vi "Termo_1.5__.vi"() -> ()   [LabVIEW 2015]
doc: "Программа мониторинга температуры"
uses:
  <vilib>/Utility/error.llb/DialogType.ctl
  Load and Save Controls_LV2009.llb/RWC_Actions.ctl
panel:
  out "?":bool
  out "graph_update":bool
  out "Конфиг. АЦП?":bool
  in  "Tab Control":enum32{"ИЗМЕРЕНИЯ [К]", " АЦП", "ГРАФИК"}(tab)
  in  "T2_visible":bool=TRUE
  out "T6":dbl format="%.2f"
  in  "T5_visible":bool=TRUE
  out "R5":dbl format="%.2f"
  out "T5":dbl format="%.2f"
  out "R1":dbl format="%.2f"
  out "T1":dbl format="%.2f"
  out "T3":dbl format="%.2f"
  out "R3":dbl format="%.2f"
  out "Alarm":bool
  out "разница Т":dbl format="%.2f"
  out "T2":dbl format="%.2f"
  out "T4":dbl format="%.2f"
  out "R2":dbl format="%.2f"
  out "R4":dbl format="%.2f"
  out "R6":dbl format="%.2f"
  in  "T1_visible":bool=TRUE
  in  "T3_visible":bool=TRUE
  in  "T4_visible":bool=TRUE
  in  "T6_visible":bool=TRUE
  in  "stop":bool
  in  "ADC_dyn_range":T1(ring)=enum."± 0.625 В"
  in  "Buf_size":u8=1 min=1 max=128
  in  "SPS":T2(ring)
  in  "IP-адрес":string="192.168.127.252"
  in  "порт":u16=4001
  in  "Очистить график":bool
  in  "load_coeff.":bool caption="Disconn"
  in  "save_coeff.":bool caption="Disconn"
  in  "Coeff_cl_ch5":T3={"k1"=19.4736079181311652, "k2"=-232.79779903171584, "k3"=1229.13228608109057005, "k4"=-3103.0388431325554801, "k5"=4219.3520172238349901, "k6"=-2697.7160155214369299, "k7"=779.55193291697651198} caption="Канал 5" {"k7" format="%#_16g"; "k6" format="%#_16g"; "k5" format="%#_16g"; "k4" format="%#_16g"; "k3" format="%#_16g"; "k2" format="%#_16g"; "k1" format="%#_16g"}
  in  "Coeff_cl_ch4":T3={"k1"=24.218377729237545301, "k2"=-311.679773783311248, "k3"=1734.44359050504863, "k4"=-4665.87189712375402, "k5"=6719.3289510309696202, "k6"=-4578.02570509165525, "k7"=1400.00134176202118} caption="Канал 4" {"k7" format="%#_16g"; "k6" format="%#_16g"; "k5" format="%#_16g"; "k4" format="%#_16g"; "k3" format="%#_16g"; "k2" format="%#_16g"; "k1" format="%#_16g"}
  in  "Coeff_cl_ch3":T3={"k1"=8.756, "k2"=-142.210000000000000006, "k3"=1253.0, "k4"=-4877.1, "k5"=10581.0, "k6"=-10354.0, "k7"=3998.5} caption="Канал 3" {"k7" format="%#_16g"; "k6" format="%#_16g"; "k5" format="%#_16g"; "k4" format="%#_16g"; "k3" format="%#_16g"; "k2" format="%#_16g"; "k1" format="%#_16g"}
  in  "Coeff_cl_ch2":T3={"k1"=31.9101907935109921, "k2"=-399.867376562207937, "k3"=2119.32627579197288, "k4"=-5531.15447566658258, "k5"=7772.21873644739389, "k6"=-5292.23886113613844, "k7"=1613.2211984321475} caption="Канал 2" {"k7" format="%#_16g"; "k6" format="%#_16g"; "k5" format="%#_16g"; "k4" format="%#_16g"; "k3" format="%#_16g"; "k2" format="%#_16g"; "k1" format="%#_16g"}
  in  "Coeff_cl_ch6":T3={"k1"=11.9061392787261866, "k2"=-139.902402561856434, "k3"=774.882810204289854, "k4"=-1837.4832512177527, "k5"=2139.5822282396256899, "k6"=-730.555961686186492, "k7"=169.810834781266749} caption="Канал 6" {"k7" format="%#_16g"; "k6" format="%#_16g"; "k5" format="%#_16g"; "k4" format="%#_16g"; "k3" format="%#_16g"; "k2" format="%#_16g"; "k1" format="%#_16g"}
  in  "GraphLookB":bool
  in  "xScale -":bool
  in  "xScale +":bool
  out "мин.":string="1"
  in  "Старт измер.":bool
  in  "Стоп измер.":bool
  in  "Добавить время":dbl(ring)=300.0 items=["10 сек."=10.0, "1 мин."=60.0, "5 мин."=300.0, "20 мин."=1200.0]
  in  "Т min":dbl=4.0 min=-10.0 max=350.0 step=0.1
  in  "Т max":dbl=300.0 min=2.0 max=500.0 step=0.1
  out "часы":string="0"
  in  "Autoscale":bool=TRUE
  out "сек.":string="0"
  out "Сутки":string
  out "счетчик":u32=4001
  in  "Запись в файл":bool
  out "Path":string
  out "refnum out":refnum<file>
  in  "header?":bool caption="Disconn"
  out "con ID":refnum<k5>
  out "Graphs T":dynamicdata(graph) caption="ТЕМПЕРАТУРА, К"
  out "Расположение файла":path
  # "Конец  соленоида"
  # "Середина\n соленоида"
  # "Перемычка"
  # "Кольцо\n спаев 1"
  # "Кольцо\n спаев 2"
  # "Шина"
  # "Конец сол/спаи dT:"
  # "Больше 40 К ?"
  # "Сопротивление, Ом"
  # "Конец соленоида"
  # "Сер. соленоида"
  # "Перемычка"
  # "1"
  # "Кольцо спаев"
  # "2"
  # "Шина"
  # "Скорость измерений"
  # "SPS = Samples Per Second"
  # "Размер буфера усреднения"
  # "Подключение"
  # "Шкала Т"
  # "Время графика"
  # ":"
  # ":"
  # "Измерения"
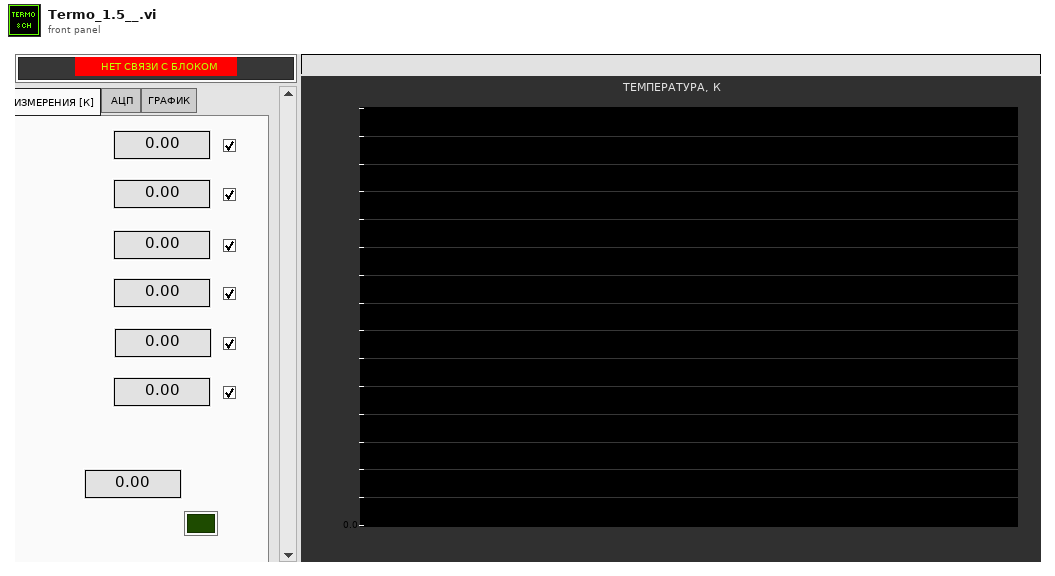
[diagram p1: front panel]
types:
  T1 = enum16{"± 5 В", "± 2.5 В", "± 1.25 В", "± 0.625 В", "± 312.5 мВ", "± 156.25 мВ", "± 78.125 мВ"}
  T2 = enum16{"2,5 SPS", "5 SPS", "10 SPS", "25 SPS", "50 SPS", "100 SPS", "500 SPS"}
  T3 = cluster{"k1":ext, "k2":ext, "k3":ext, "k4":ext, "k5":ext, "k6":ext, "k7":ext}
  T4 = typedef "RWC_Actions.ctl" = enum16{"Read", "Write", "Read and Create"}
  T5 = typedef "DialogType.ctl" = u16
  T6 = enum32{"Page Enabled", "Page Disabled", "Page Disabled & Grayed"}
  T7 = enum16{"Standard", "Buffered", "CRLF", "Immediate"}
  T8 = cluster{" T1":dbl, "T2":dbl, "T3":dbl, "T4":dbl, " T5":dbl, "T6":dbl}
  T9 = typedef "LVDateTimeRec.ctl" = cluster{"fractional second":dbl, "second":i32, "minute":i32, "hour":i32, "day of month":i32, "month":i32, "year":i32, "day of week":i32, "day of year":i32, "DST":i32}
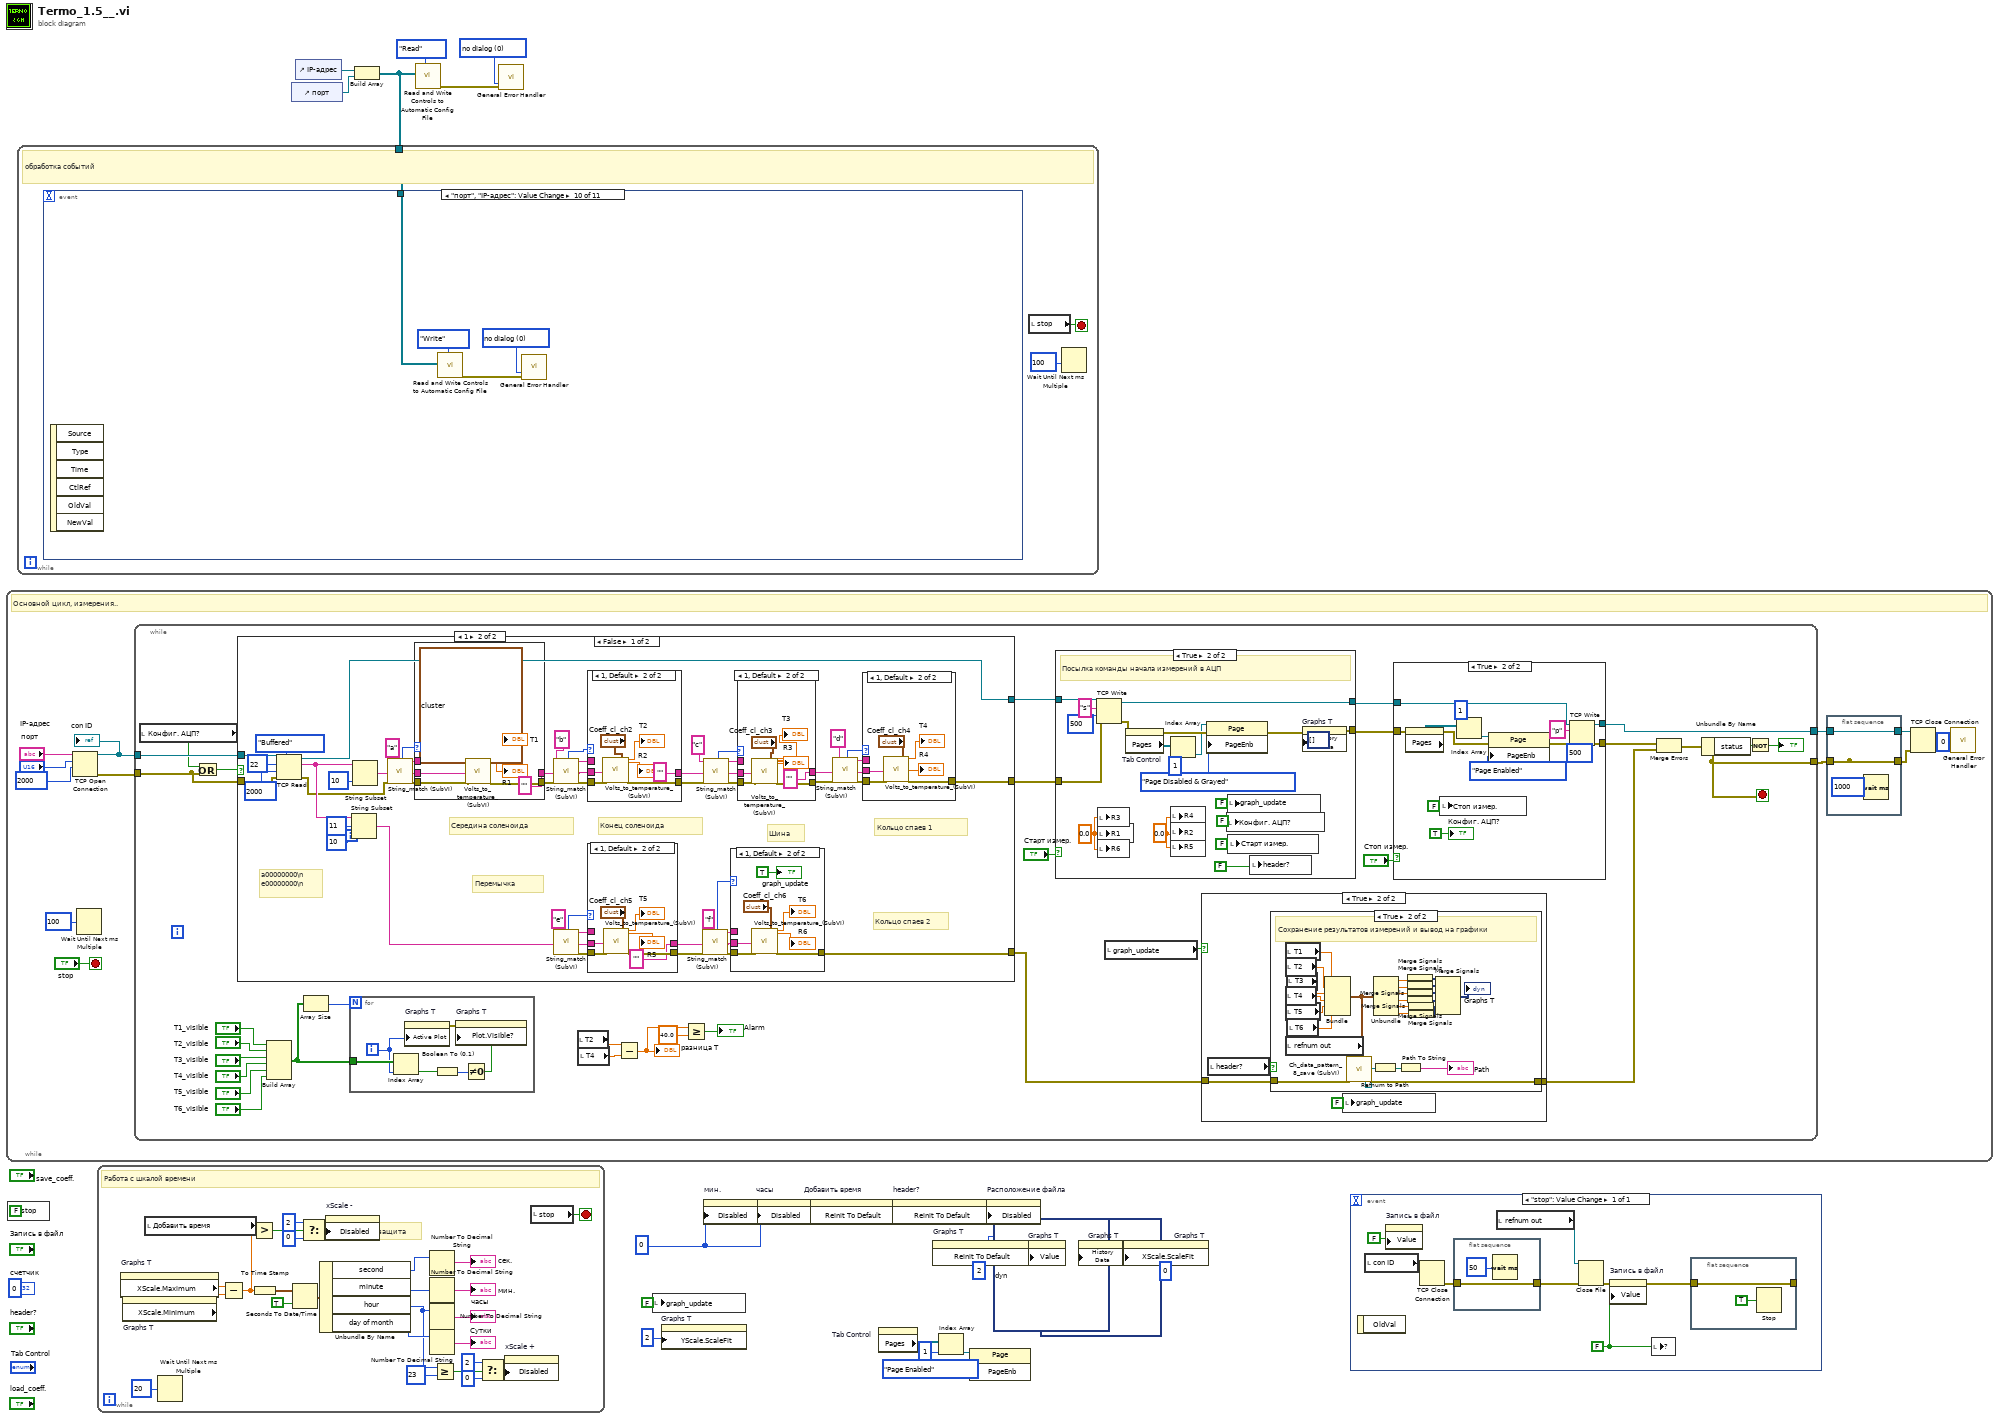
[diagram p0: block diagram]
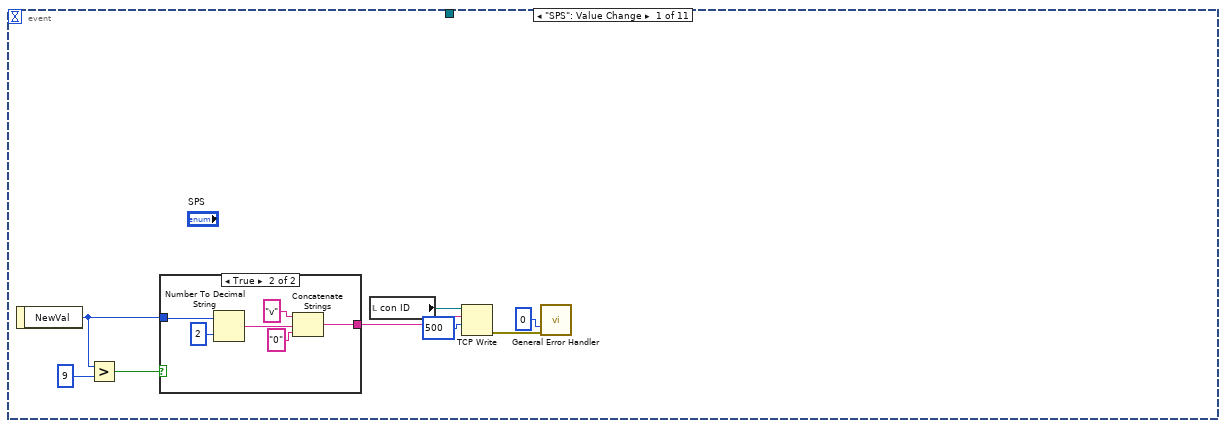
[diagram p2: hidden frame]
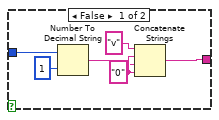
[diagram p3: hidden frame]
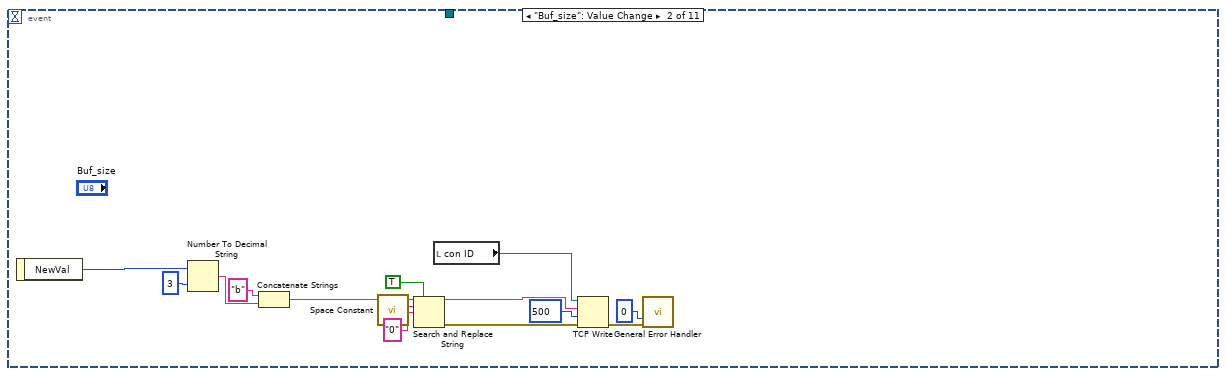
[diagram p4: hidden frame]
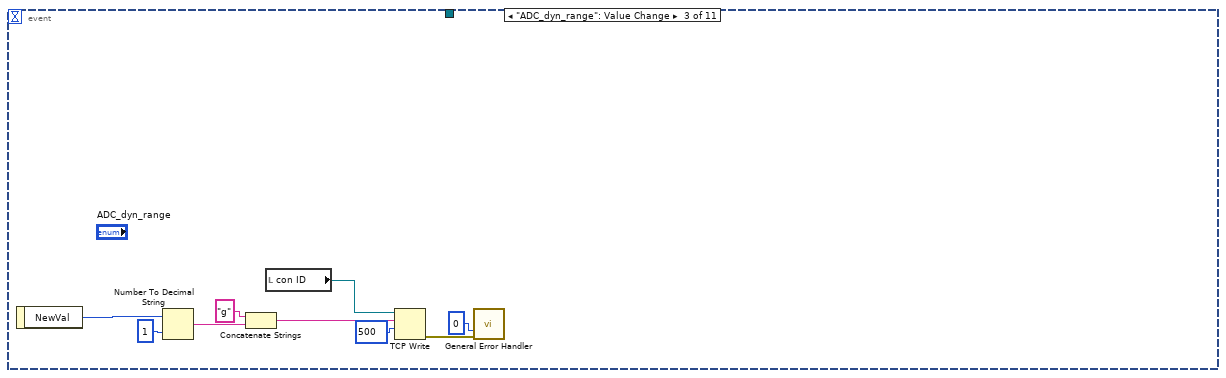
[diagram p5: hidden frame]
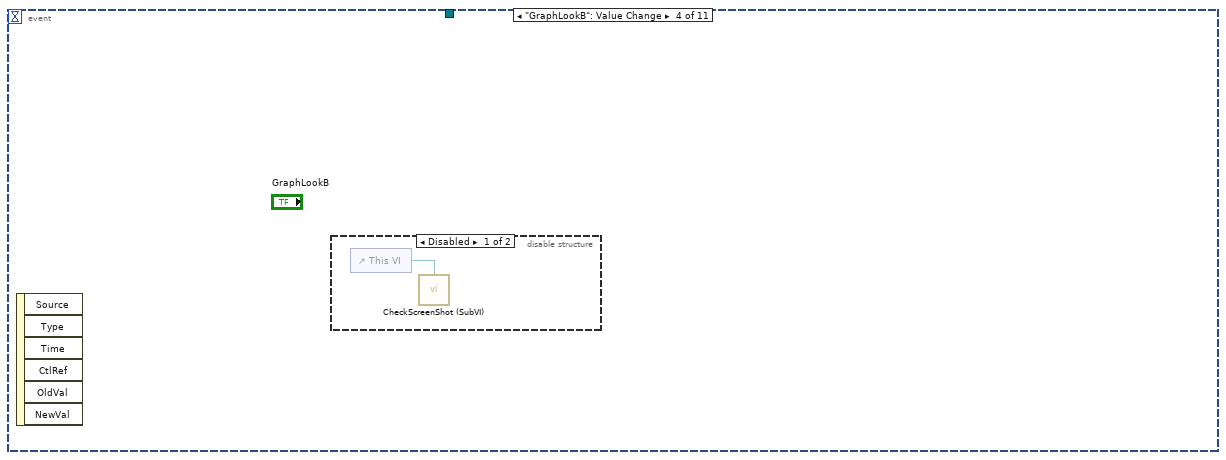
[diagram p6: hidden frame]
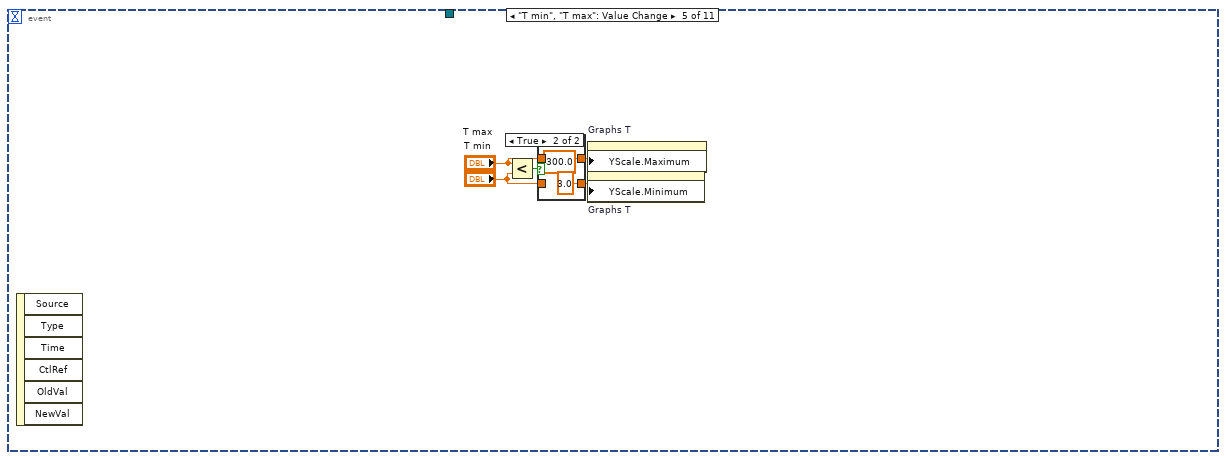
[diagram p8: hidden frame]
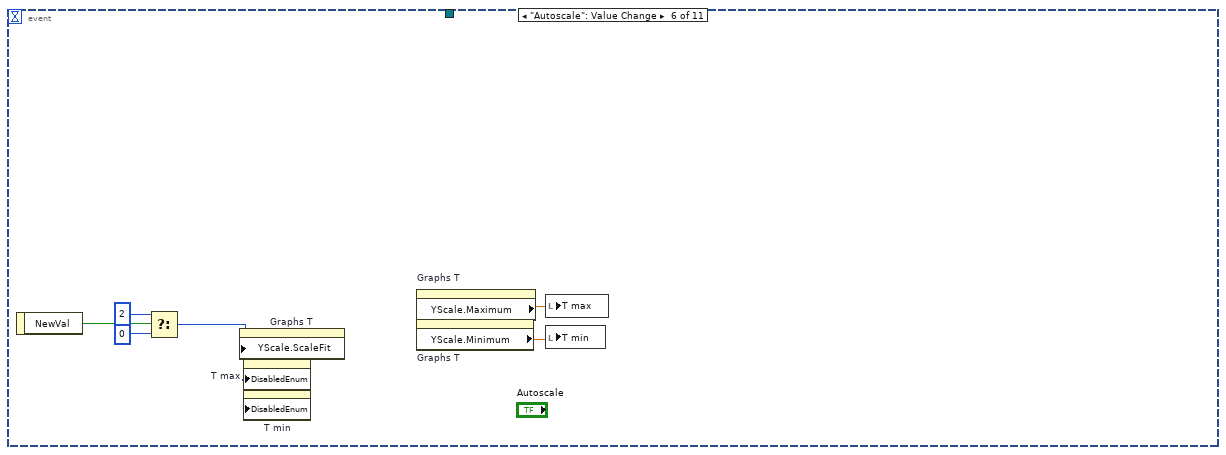
[diagram p10: hidden frame]
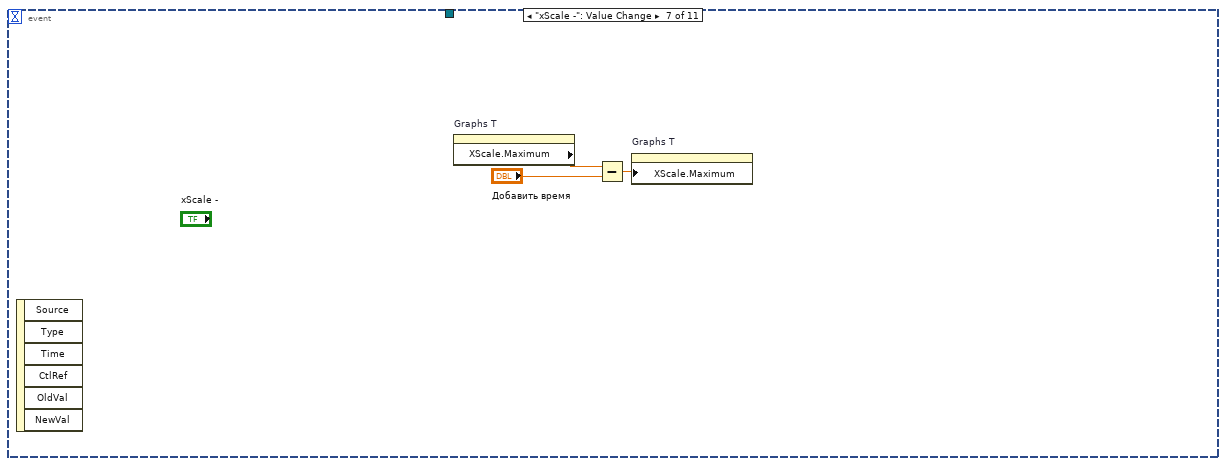
[diagram p11: hidden frame]
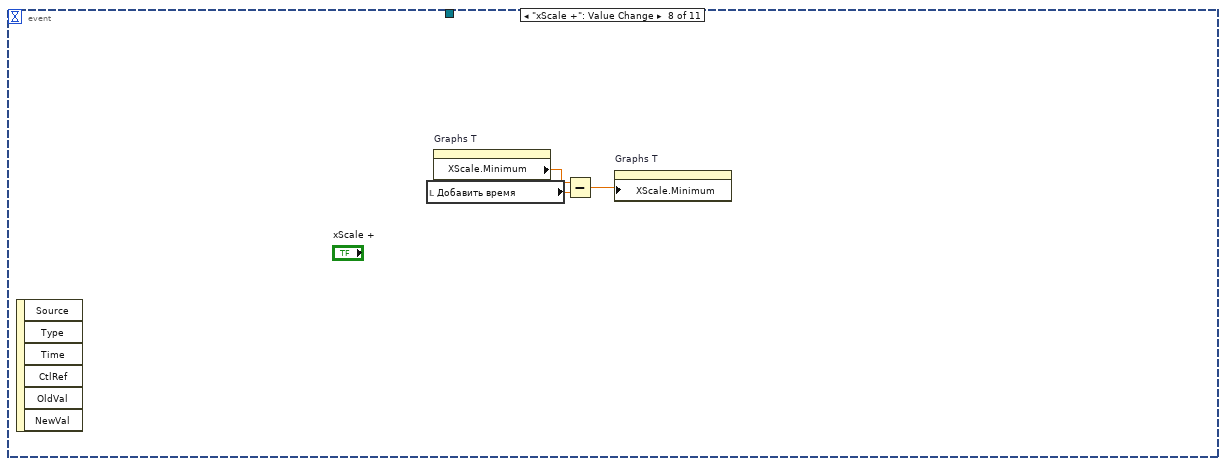
[diagram p12: hidden frame]
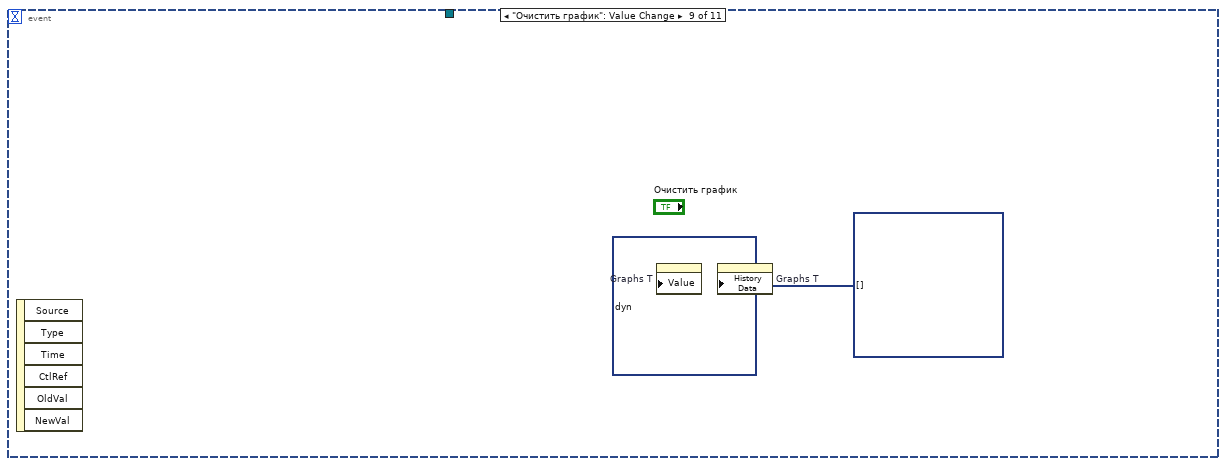
[diagram p13: hidden frame]
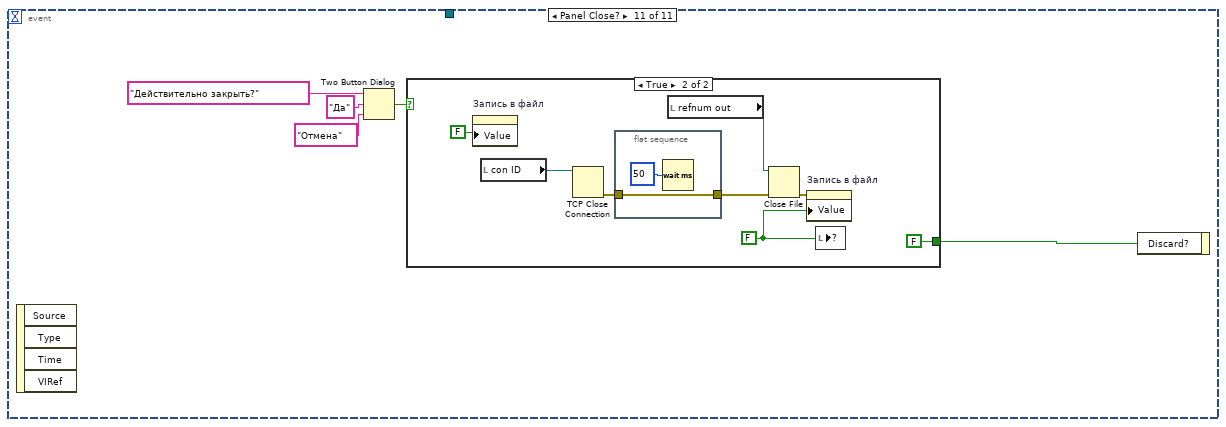
[diagram p14: hidden frame]
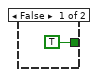
[diagram p15: hidden frame]
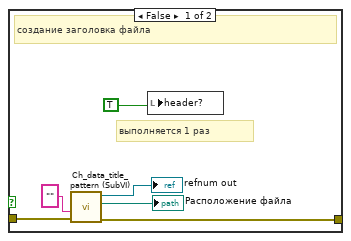
[diagram p17: hidden frame]
diagram:
  w6 = T5 0 items=["no dialog", "OK message", "continue or stop message", "OK message + warnings", "continue/stop + warnings"] ("type of dialog (OK msg:1)")
  w25 = u8 0 ("Disabled")
  n1 = while {
    stop <- "stop" stop-if-true
    # "Основной цикл, измерения.."
    n2 = TCP Open Connection(address="IP-адрес", remote port or service name="порт", timeout ms (60000)=2000) -> (connection ID=w38:refnum<k5>, error out=w32:errorcluster)  [unwired: 1 in, 1 out]
    "con ID" <- w38
    n3 = Wait Until Next ms Multiple(millisecond multiple=u32 100) -> ()  [unwired: 1 out]
    n4 = while {
      tunnel: w38 -> [w73]
      tunnel: w32 -> [w51]
      tunnel: [w44] -> w30
      tunnel: [w43] -> w28
      stop <- w43 stop-if-true
      n5 = local read "Конфиг. АЦП?"() -> (w52:bool)
      n6 = Or(x=w52, y=w51) -> (x .or. y?=w66:bool)
      n7 = case shown="False" w66 {
        tunnel: [w156 w259] -> w53
        tunnel: w73 -> [w159 w259]
        tunnel: [w155 w258] -> w49
        tunnel: w51 -> [w157 w258]
        tunnel: [w154 _] -> w47
        frame False {
          # "a00000000\\n\ne00000000\\n"
          # "Кольцо спаев 2"
          # "Шина"
          # "Перемычка"
          # "Кольцо спаев 1"
          # "Конец соленоида"
          # "Середина соленоида"
          n8 = TCP Read(connection ID=w159, bytes to read=22, error in (no error)=w157, 7:T7."Buffered" ("mode (standard)"), 9:2000 ("timeout ms (25000)")) -> (connection ID out=w156:refnum<k5>, data out=w163:string, error out=w158:errorcluster)
          n9 = String Subset(string=w163, offset (0)=11, length (rest)=10 ("length (rest)")) -> (substring=w160:string)
          n10 = String Subset(string=w163, length (rest)=10 ("length (rest)")) -> (substring=w165:string)  [unwired: 1 in]
          n11 = call "String_match (SubVI).vi"("channel id"="a" ("regular expression"), "input string"=w165, "error in"=w158) -> ("match ?"=w171:i32, "output string"=w199:string, "match substring"=w200:string, "error out"=w201:errorcluster)  [unwired: 13 in]
          n12 = case shown="1" w171 {
            tunnel: [w250 w256] -> w190
            tunnel: w201 -> [w250 w257]
            tunnel: w200 -> [_ w252]
            tunnel: [w249 "" ("output string")] -> w203
            tunnel: w199 -> [w249 _]
            frame -1, Default {
            }
            frame 1 {
              n13 = call "Volts_to_temperature_(SubVI).vi"("ch_data_string"=w252, "error in"=w257, "koeff. cluster"=T3 {"k1"=20.678416953771299999, "k2"=-270.806564304511, "k3"=1559.71508308313, "k4"=-4317.07993103563, "k5"=6444.9990497231400002, "k6"=-4562.30018320679, "k7"=1455.99202726967}) -> ("T solvation"=→"T1":dbl, "meas_voltage"=→"R1":dbl, "error out"=w256:errorcluster)  [unwired: 20 in, 2 out]
            }
          }
          n14 = call "String_match (SubVI).vi"("channel id"="b" ("regular expression"), "input string"=w203, "error in"=w190) -> ("match ?"=w170:i32, "output string"=w195:string, "match substring"=w196:string, "error out"=w197:errorcluster)  [unwired: 13 in]
          n15 = call "String_match (SubVI).vi"("channel id"="e" ("regular expression"), "input string"=w160) -> ("match ?"=w167:i32, "output string"=w188:string, "match substring"=w187:string, "error out"=w186:errorcluster)  [unwired: 14 in]
          n16 = case shown="1, Default" w170 {
            tunnel: [w241 w248] -> w179
            tunnel: w197 -> [w241 w247]
            tunnel: w196 -> [_ w246]
            tunnel: w195 -> [w240 _]
            tunnel: [w240 "" ("output string")] -> w178
            frame -1 {
            }
            frame 1, Default {
              n17 = call "Volts_to_temperature_(SubVI).vi"("ch_data_string"=w246, "error in"=w247, "koeff. cluster"="Coeff_cl_ch2") -> ("T solvation"=→"T2":dbl, "meas_voltage"=→"R2":dbl, "error out"=w248:errorcluster)  [unwired: 20 in, 2 out]
            }
          }
          n18 = case shown="1, Default" w167 {
            tunnel: [w225 w232] -> w189
            tunnel: w186 -> [w225 w231]
            tunnel: w187 -> [_ w230]
            tunnel: [w224 "" ("output string")] -> w184
            tunnel: w188 -> [w224 _]
            frame -1 {
            }
            frame 1, Default {
              n19 = call "Volts_to_temperature_(SubVI).vi"("ch_data_string"=w230, "error in"=w231, "koeff. cluster"="Coeff_cl_ch5") -> ("T solvation"=→"T5":dbl, "meas_voltage"=→"R5":dbl, "error out"=w232:errorcluster)  [unwired: 20 in, 2 out]
            }
          }
          n20 = call "String_match (SubVI).vi"("channel id"="f" ("regular expression"), "input string"=w184, "error in"=w189) -> ("match ?"=w166:i32, "output string"=w183:string, "match substring"=w182:string, "error out"=w181:errorcluster)  [unwired: 13 in]
          n21 = call "String_match (SubVI).vi"("channel id"="c" ("regular expression"), "input string"=w178, "error in"=w179) -> ("match ?"=w169:i32, "output string"=w174:string, "match substring"=w175:string, "error out"=w176:errorcluster)  [unwired: 13 in]
          n22 = case shown="1, Default" w166 {
            tunnel: [w216 w223] -> w154
            tunnel: w181 -> [w216 w222]
            tunnel: w182 -> [_ w221]
            tunnel: w183 -> [_ _]
            frame -1 {
            }
            frame 1, Default {
              n23 = call "Volts_to_temperature_(SubVI).vi"("ch_data_string"=w221, "error in"=w222, "koeff. cluster"="Coeff_cl_ch6") -> ("T solvation"=→"T6":dbl, "meas_voltage"=→"R6":dbl, "error out"=w223:errorcluster)  [unwired: 20 in, 2 out]
              "graph_update" <- TRUE ("graph_update")
            }
          }
          n24 = case shown="1, Default" w169 {
            tunnel: w176 -> [w208 w214]
            tunnel: [w208 w213] -> w173
            tunnel: w175 -> [_ w210]
            tunnel: w174 -> [w207 _]
            tunnel: [w207 "" ("output string")] -> w172
            frame -1 {
            }
            frame 1, Default {
              n25 = call "Volts_to_temperature_(SubVI).vi"("ch_data_string"=w210, "error in"=w214, "koeff. cluster"="Coeff_cl_ch3") -> ("T solvation"=→"T3":dbl, "meas_voltage"=→"R3":dbl, "error out"=w213:errorcluster)  [unwired: 20 in, 2 out]
            }
          }
          n26 = call "String_match (SubVI).vi"("channel id"="d" ("regular expression"), "input string"=w172, "error in"=w173) -> ("match ?"=w168:i32, "output string"=w191:string, "match substring"=w192:string, "error out"=w193:errorcluster)  [unwired: 13 in]
          n27 = case shown="1, Default" w168 {
            tunnel: w193 -> [w233 w239]
            tunnel: [w233 w238] -> w155
            tunnel: w192 -> [_ w236]
            tunnel: w191 -> [_ _]
            frame -1 {
            }
            frame 1, Default {
              n28 = call "Volts_to_temperature_(SubVI).vi"("ch_data_string"=w236, "error in"=w239, "koeff. cluster"="Coeff_cl_ch4") -> ("T solvation"=→"T4":dbl, "meas_voltage"=→"R4":dbl, "error out"=w238:errorcluster)  [unwired: 20 in, 2 out]
            }
          }
        }
        frame True {
        }
      }
      n29 = Build Array("T1_visible", "T2_visible", "T3_visible", "T4_visible", "T5_visible", "T6_visible") -> (w58:bool[])
      n30 = Array Size(array=w58) -> (size(s)=w59:i32)
      n31 = for {
        N: w59 -> [_]
        tunnel: w58 -> [w152]
        i -> [w150]
        n32 = Index Array(array=w152, index=w150) -> (element=w149:bool)
        n33 = property on="Graphs T" class="WFChart (strict)"("Active Plot"=w150) -> (error out=w151:errorcluster)  [unwired: 2 in, 1 out]
        n34 = Boolean To (0,1)(Boolean=w149) -> (0, 1=w153:i16)
        n35 = Not Equal To 0?(x=w153) -> (x != 0?=w148:bool)
        n36 = property on="Graphs T" class="WFChart (strict)"(error in=w151, "Plot.Visible?"=w148) -> ()  [unwired: 1 in, 2 out]
      }
      n37 = local read "T2"() -> (w68:dbl)
      n38 = local read "T4"() -> (w67:dbl)
      n39 = Subtract(x=w68, y=w67) -> (x-y=w69:dbl)
      "разница Т" <- w69
      n40 = Greater Or Equal?(x=w69, y=40.0) -> (x >= y?=→"Alarm":bool)
      n41 = case shown="True" "Старт измер." {
        tunnel: [w126 w137] -> w55
        tunnel: [w127 w136] -> w57
        tunnel: w53 -> [w127 w131]
        tunnel: w49 -> [w126 w130]
        frame False {
        }
        frame True {
          w133 = 0.0 ("3")
          w128 = 0.0 ("3")
          # "Посылка команды начала измерений в АЦП"
          n42 = TCP Write(connection ID=w131, data in="s", error in (no error)=w130, 9:500 ("timeout ms (25000)")) -> (connection ID out=w136:refnum<k5>, error out=w145:errorcluster)  [unwired: 1 out]
          n43 = local write "R3"(w128) -> ()
          n44 = local write "R1"(w128) -> ()
          n45 = local write "R6"(w128) -> ()
          n46 = property on="Tab Control" class="TabCtl (strict)"(error in=w145) -> (error out=w146:errorcluster, "Pages"=w141:refnum<vi>[])  [unwired: 1 in, 1 out]
          n47 = Index Array(array=w141, index=1) -> (element=w142:refnum<vi>)
          n48 = local write "R4"(w133) -> ()
          n49 = local write "R2"(w133) -> ()
          n50 = local write "R5"(w133) -> ()
          n51 = property class="Page"(reference=w142, error in=w146, "PageEnb"=T6."Page Disabled & Grayed" ("Page Enabled State")) -> (error out=w132:errorcluster)  [unwired: 1 out]
          n52 = local write "Конфиг. АЦП?"(FALSE ("Старт измер.")) -> ()
          n53 = local write "graph_update"(FALSE ("graph_update")) -> ()
          n54 = local write "Старт измер."(FALSE ("Старт измер.")) -> ()
          n55 = local write "header?"(FALSE ("flag1")) -> ()
          n56 = property on="Graphs T" class="WFChart (strict)"(error in=w132, "History Data"=dynamicdata[] []) -> (error out=w137:errorcluster)  [unwired: 1 in, 1 out]
        }
      }
      n57 = local read "graph_update"() -> (w48:bool)
      n58 = case shown="True" w48 {
        tunnel: w47 -> [w74 w76]
        tunnel: [w74 w75] -> w45
        frame False {
        }
        frame True {
          n59 = local read "header?"() -> (w78:bool)
          n60 = case shown="True" w78 {
            tunnel: w76 -> [w79 w87]
            tunnel: [w81 w86] -> w75
            frame False {
              # "выполняется 1 раз"
              # "создание заголовка файла"
              n61 = call "Ch_data_title_pattern (SubVI).vi"("error in"=w79, "Единица измерений"="") -> ("error out"=w81:errorcluster, "Path"=→"Расположение файла":path, "Byte Stream File out"=→"refnum out":refnum<file>)  [unwired: 7 in]
              n62 = local write "header?"(TRUE ("flag1")) -> ()
            }
            frame True {
              # "Сохранение результатов измерений и вывод на графики"
              n63 = local read "T1"() -> (w109:dbl)
              n64 = local read "T2"() -> (w108:dbl)
              n65 = local read "T4"() -> (w94:dbl)
              n66 = local read "T5"() -> (w93:dbl)
              n67 = local read "refnum out"() -> (w85:refnum<file>)
              n68 = local read "T3"() -> (w95:dbl)
              n69 = local read "T6"() -> (w90:dbl)
              n70 = Bundle("T1"=w109, "T2"=w108, "T3"=w95, "T4"=w94, "T5"=w93, "T6"=w90) -> (w107:T8)  [unwired: 1 in]
              n71 = call "Ch_data_pattern_8_save (SubVI).vi"("error in"=w87, "T Cluster"=w107, "file"=w85) -> ("error out"=w86:errorcluster)  [unwired: 24 in]
              n72 = Refnum to Path(1:w85) -> (0:w106:path)
              n73 = Unbundle(w107) -> ("T1"=w99:dbl, "T2"=w98:dbl, "T3"=w97:dbl, "T4"=w96:dbl, "T5"=w91:dbl, "T6"=w88:dbl)
              n74 = Path To String(path=w106) -> (string=→"Path":string)
              n75 = Merge Signals(w99) -> (w102:dynamicdata)
              n76 = Merge Signals(w98) -> (w103:dynamicdata)
              n77 = Merge Signals(w97) -> (w104:dynamicdata)
              n78 = Merge Signals(w96) -> (w101:dynamicdata)
              n79 = Merge Signals(w91) -> (w92:dynamicdata)
              n80 = Merge Signals(w88) -> (w89:dynamicdata)
              n81 = Merge Signals(w102, w103, w104, w101, w92, w89) -> (→"Graphs T":dynamicdata)
            }
          }
          n82 = local write "graph_update"(FALSE ("graph_update")) -> ()
        }
      }
      n83 = case shown="True" "Стоп измер." {
        tunnel: w55 -> [w110 w118]
        tunnel: w57 -> [w111 w116]
        tunnel: [w110 w112] -> w46
        tunnel: [w111 w113] -> w44
        frame False {
        }
        frame True {
          n84 = property on="Tab Control" class="TabCtl (strict)"(error in=w118) -> (error out=w117:errorcluster, "Pages"=w121:refnum<vi>[])  [unwired: 1 in, 1 out]
          n85 = local write "Стоп измер."(FALSE ("Стоп измер.")) -> ()
          n86 = Index Array(array=w121, index=1) -> (element=w122:refnum<vi>)
          n87 = property class="Page"(reference=w122, error in=w117, "PageEnb"=T6."Page Enabled" ("Page Enabled State")) -> (error out=w125:errorcluster)  [unwired: 1 out]
          n88 = TCP Write(connection ID=w116, data in="p", error in (no error)=w125, 9:500 ("timeout ms (25000)")) -> (connection ID out=w113:refnum<k5>, error out=w112:errorcluster)  [unwired: 1 out]
          "Конфиг. АЦП?" <- TRUE ("Конфиг. АЦП?")
        }
      }
      n89 = Merge Errors(w46, w45) -> (w43:errorcluster)
      n90 = Unbundle By Name(w43) -> ("status"=w50:bool)
      n91 = Not(x=w50) -> (.not. x?=→"?":bool)
    }
    n92 = flat-sequence {
      tunnel: [w41] -> w29
      tunnel: w30 -> [w41]
      tunnel: w28 -> [w40]
      tunnel: [w40] -> _
      tunnel: [w40] -> w27
      frame #0 {
        n93 = Wait (ms)(milliseconds to wait=u32 1000) -> ()  [unwired: 1 out]
      }
    }
    n94 = TCP Close Connection(connection ID=w29, error in (no error)=w27) -> (error out=w37:errorcluster)  [unwired: 2 out]
    n95 = call <vilib>:"General Error Handler.vi"("type of dialog (OK msg:1)"=u32 0 ("milliseconds to wait"), "error in (no error)"=w37) -> ()  [unwired: 1 in, 13 out]
  }
  n96 = local write "stop"(FALSE ("Boolean")) -> ()
  n97 = while {
    stop <- w285 stop-if-true
    # "защита"
    # "Работа с шкалой времени"
    n98 = property on="Graphs T" class="WFChart (strict)"() -> ("XScale.Maximum"=w261:dbl)  [unwired: 2 in, 2 out]
    n99 = property on="Graphs T" class="WFChart (strict)"() -> ("XScale.Minimum"=w260:dbl)  [unwired: 2 in, 2 out]
    n100 = local read "Добавить время"() -> (w284:dbl)
    n101 = Wait Until Next ms Multiple(millisecond multiple=u32 20) -> ()  [unwired: 1 out]
    n102 = Subtract(x=w261, y=w260) -> (x-y=w274:dbl)
    n103 = Greater?(x=w284, y=w274) -> (0:w267:bool)
    n104 = To Time Stamp(1:w274) -> (0:w282:timestamp)
    n105 = Seconds To Date/Time(time stamp (now)=w282, to UTC (F)=TRUE) -> (date time rec=w281:T9)
    n106 = Select(t=u8 2 ("Disabled"), s=w267, f=u8 0 ("Disabled")) -> (s? t:f=w270:u8)
    n107 = Unbundle By Name(w281) -> ("second"=w280:i32, "minute"=w279:i32, "hour"=w272:i32, "day of month"=w278:i32)
    n108 = property on="xScale -" class="Bool (strict)"("Disabled"=w270) -> ()  [unwired: 2 in, 2 out]
    n109 = Number To Decimal String(number=w280) -> (decimal integer string=→"сек.":string)  [unwired: 1 out]
    n110 = Number To Decimal String(number=w279) -> (decimal integer string=→"мин.":string)  [unwired: 1 out]
    n111 = Number To Decimal String(number=w272) -> (decimal integer string=→"часы":string)  [unwired: 1 out]
    n112 = Number To Decimal String(number=w278) -> (decimal integer string=→"Сутки":string)  [unwired: 1 out]
    n113 = Greater Or Equal?(x=w272, y=23) -> (x >= y?=w263:bool)
    n114 = Select(t=u8 2 ("Disabled"), s=w263, f=u8 0 ("Disabled")) -> (s? t:f=w266:u8)
    n115 = property on="xScale +" class="Bool (strict)"("Disabled"=w266) -> ()  [unwired: 2 in, 2 out]
    n116 = local read "stop"() -> (w285:bool)
  }
  n117 = control-ref of="порт"() -> (w2:refnum<vi>)
  n118 = control-ref of="IP-адрес"() -> (w3:refnum<vi>)
  n119 = Build Array(w3, w2) -> (w1:refnum<vi>[])
  n120 = while {
    tunnel: w1 -> [w286]
    stop <- w287 stop-if-true
    # "обработка событий"
    n121 = event shown="[9] \"порт\", \"IP-адрес\": Value Change" {
      selector: _ -> [_ _ _ _ _ _ _ _ _ _ _]
      dyn-events: _ -> [_ _ _ _ _ _ _ _ _ _ _]
      timeout: _ -> [_ _ _ _ _ _ _ _ _ _ _]
      tunnel: w286 -> [_ _ _ _ _ _ _ _ _ w357 _]
      event "SPS": Value Change {
        n122 = event-data() -> ("NewVal"=w292:T2)  [unwired: 1 in]
        n123 = Greater?(x=w292, y=9 ("timeout ms (25000)")) -> (0:w290:bool)
        n124 = case shown="True" w290 {
          tunnel: w292 -> [w302 w308]
          tunnel: [w299 w303] -> w289
          frame False {
            w298 = "0" ("string")
            n125 = Number To Decimal String(number=w302, width (-)=i16 1) -> (decimal integer string=w297:string)
            n126 = Concatenate Strings("v" ("data in"), w298, w297, w298) -> (w299:string)
          }
          frame True {
            n127 = Number To Decimal String(number=w308, width (-)=i16 2) -> (decimal integer string=w305:string)
            n128 = Concatenate Strings("v" ("data in"), w305, "0" ("string")) -> (w303:string)
          }
        }
        n129 = local read "con ID"() -> (w295:refnum<k5>)
        n130 = TCP Write(connection ID=w295, data in=w289, 9:500 ("timeout ms (25000)")) -> (error out=w294:errorcluster)  [unwired: 1 in, 2 out]
        n131 = call <vilib>:"General Error Handler.vi"("type of dialog (OK msg:1)"=0 ("timeout ms (25000)"), "error in (no error)"=w294) -> ()  [unwired: 9 in, 5 out]
      }
      event "Buf_size": Value Change {
        n132 = event-data() -> ("NewVal"=w319:u8)  [unwired: 1 in]
        n133 = Number To Decimal String(number=w319, width (-)=i16 3) -> (decimal integer string=w317:string)
        n134 = Concatenate Strings("b" ("data in"), w317) -> (w316:string)
        n135 = call <vilib>:"Space Constant.vi"() -> ("String"=w314:string)
        n136 = Search and Replace String(replace all?=TRUE ("replace all? (F)"), input string=w316, search string=w314, replace string="0" ("replace string (\"\")")) -> (result string=w315:string, error out=w311:errorcluster)  [unwired: 4 in, 2 out]
        n137 = local read "con ID"() -> (w321:refnum<k5>)
        n138 = TCP Write(connection ID=w321, data in=w315, error in (no error)=w311, 9:500 ("timeout ms (25000)")) -> (error out=w310:errorcluster)  [unwired: 2 out]
        n139 = call <vilib>:"General Error Handler.vi"("type of dialog (OK msg:1)"=0 ("timeout ms (25000)"), "error in (no error)"=w310) -> ()  [unwired: 9 in, 5 out]
      }
      event "ADC_dyn_range": Value Change {
        n140 = event-data() -> ("NewVal"=w328:T1)  [unwired: 1 in]
        n141 = Number To Decimal String(number=w328, width (-)=i16 1) -> (decimal integer string=w326:string)
        n142 = Concatenate Strings("g" ("data in"), w326) -> (w325:string)
        n143 = local read "con ID"() -> (w330:refnum<k5>)
        n144 = TCP Write(connection ID=w330, data in=w325, 9:500 ("timeout ms (25000)")) -> (error out=w323:errorcluster)  [unwired: 1 in, 2 out]
        n145 = call <vilib>:"General Error Handler.vi"("type of dialog (OK msg:1)"=0 ("timeout ms (25000)"), "error in (no error)"=w323) -> ()  [unwired: 9 in, 5 out]
      }
      event "GraphLookB": Value Change {
        n146 = event-data() -> ()  [unwired: 1 in, 6 out]
        n147 = disable-structure shown="Disabled" {
          frame Disabled {
            n148 = control-ref of="This VI"() -> (w332:refnum<vi>)
            n149 = call "CheckScreenShot (SubVI).vi"("VI reference"=w332) -> ()  [unwired: 15 in]
          }
          frame Enabled {
          }
        }
      }
      event "Т min", "Т max": Value Change {
        n150 = event-data() -> ()  [unwired: 1 in, 6 out]
        n151 = Less?(x="Т max", y="Т min") -> (x < y?=w333:bool)
        n152 = case shown="True" w333 {
          tunnel: [w338 300.0 ("x+1")] -> w335
          tunnel: [w339 3.0 ("x+1")] -> w334
          tunnel: "Т max" -> [w338 _]
          tunnel: "Т min" -> [w339 _]
          frame False {
          }
          frame True {
          }
        }
        n153 = property on="Graphs T" class="WFChart (strict)"("YScale.Maximum"=w335) -> ()  [unwired: 2 in, 2 out]
        n154 = property on="Graphs T" class="WFChart (strict)"("YScale.Minimum"=w334) -> ()  [unwired: 2 in, 2 out]
      }
      event "Autoscale": Value Change {
        n155 = event-data() -> ("NewVal"=w342:bool)  [unwired: 1 in]
        n156 = Select(t=u8 2 ("Y Scale.Scale Fit"), s=w342, f=u8 0 ("Y Scale.Scale Fit")) -> (s? t:f=w345:u8)
        n157 = property on="Graphs T" class="WFChart (strict)"("YScale.ScaleFit"=w345) -> ()  [unwired: 2 in, 2 out]
        n158 = property on="Т max" class="DigNum (strict)"("DisabledEnum"=w345) -> ()  [unwired: 2 in, 2 out]
        n159 = property on="Т min" class="DigNum (strict)"("DisabledEnum"=w345) -> ()  [unwired: 2 in, 2 out]
        n160 = property on="Graphs T" class="WFChart (strict)"() -> ("YScale.Maximum"=w343:dbl)  [unwired: 2 in, 2 out]
        n161 = property on="Graphs T" class="WFChart (strict)"() -> ("YScale.Minimum"=w344:dbl)  [unwired: 2 in, 2 out]
        n162 = local write "Т max"(w343) -> ()
        n163 = local write "Т min"(w344) -> ()
      }
      event "xScale -": Value Change {
        n164 = event-data() -> ()  [unwired: 1 in, 6 out]
        n165 = property on="Graphs T" class="WFChart (strict)"() -> ("XScale.Maximum"=w350:dbl)  [unwired: 2 in, 2 out]
        n166 = Subtract(x=w350, y="Добавить время") -> (x-y=w349:dbl)
        n167 = property on="Graphs T" class="WFChart (strict)"("XScale.Maximum"=w349) -> ()  [unwired: 2 in, 2 out]
      }
      event "xScale +": Value Change {
        n168 = event-data() -> ()  [unwired: 1 in, 6 out]
        n169 = local read "Добавить время"() -> (w351:dbl)
        n170 = property on="Graphs T" class="WFChart (strict)"() -> ("XScale.Minimum"=w353:dbl)  [unwired: 2 in, 2 out]
        n171 = Subtract(x=w353, y=w351) -> (x-y=w352:dbl)
        n172 = property on="Graphs T" class="WFChart (strict)"("XScale.Minimum"=w352) -> ()  [unwired: 2 in, 2 out]
      }
      event "Очистить график": Value Change {
        n173 = event-data() -> ()  [unwired: 1 in, 6 out]
        n174 = property on="Graphs T" class="WFChart (strict)"("Value"=dynamicdata [{"t0"=timestamp(3465273261.7246556 s since 1904-01-01), "dt"=1.0, "Y"=[0.1931097262457384]}, {"t0"=timestamp(3465273261.7246556 s since 1904-01-01), "dt"=1.0, "Y"=[0.3594116459482981]}, {"t0"=timestamp(3465273261.7246556 s since 1904-01-01), "dt"=1.0, "Y"=[0.8898205452798131]}, {"t0"=timestamp(3465273261.7246556 s since 1904-01-01), "dt"=1.0, "Y"=[0.747699236883661]}] ("Graphs")) -> (error out=w355:errorcluster)  [unwired: 2 in, 1 out]
        n175 = property on="Graphs T" class="WFChart (strict)"(error in=w355, "History Data"=dynamicdata[] []) -> ()  [unwired: 1 in, 2 out]
      }
      event "порт", "IP-адрес": Value Change {
        w358 = T5 0 items=["no dialog", "OK message", "continue or stop message", "OK message + warnings", "continue/stop + warnings"] ("type of dialog (OK msg:1)")
        n176 = event-data() -> ()  [unwired: 1 in, 6 out]
        n177 = call "Read and Write Controls to Automatic Config File.vi"("Action"=RWC_Actions."Write", "Control References"=w357) -> ("error out"=w359:errorcluster)  [unwired: 9 in]
        n178 = call <vilib>:"General Error Handler.vi"("type of dialog (OK msg:1)"=w358, "error in (no error)"=w359) -> ()  [unwired: 1 in, 13 out]
      }
      event Panel Close? {
        n179 = event-data() -> ()  [unwired: 1 in, 4 out]
        n180 = Two Button Dialog(message="Действительно закрыть?", 1:"Отмена" ("T button name (\"OK\")"), 2:"Да" ("T button name (\"OK\")")) -> (T button?=w362:bool)
        n181 = case shown="True" w362 {
          tunnel: [TRUE ("Discard?") FALSE ("Discard?")] -> w361
          frame False {
          }
          frame True {
            w371 = FALSE ("Запись в файл")
            n182 = property on="Запись в файл" class="Bool (strict)"("Value"=FALSE ("Запись в файл")) -> ()  [unwired: 2 in, 2 out]
            n183 = local read "con ID"() -> (w368:refnum<k5>)
            n184 = TCP Close Connection(connection ID=w368) -> (error out=w374:errorcluster)  [unwired: 1 in, 2 out]
            n185 = flat-sequence {
              tunnel: [w375] -> w373
              tunnel: w374 -> [w375]
              frame #0 {
                n186 = Wait (ms)(milliseconds to wait=u32 50) -> ()  [unwired: 1 out]
              }
            }
            n187 = local read "refnum out"() -> (w370:refnum<file>)
            n188 = Close File(refnum=w370, error in=w373) -> (error out=w369:errorcluster)  [unwired: 1 out]
            n189 = property on="Запись в файл" class="Bool (strict)"(error in=w369, "Value"=w371) -> ()  [unwired: 1 in, 2 out]
            n190 = local write item#8(w371) -> ()
          }
        }
        n191 = event-data("Discard?"=w361) -> ()  [unwired: 1 in, 1 out]
      }
    }
    n192 = local read "stop"() -> (w287:bool)
    n193 = Wait Until Next ms Multiple(millisecond multiple=u32 100 ("milliseconds to wait")) -> ()  [unwired: 1 out]
  }
  n194 = call "Read and Write Controls to Automatic Config File.vi"("Action"=RWC_Actions."Read", "Control References"=w1) -> ("error out"=w5:errorcluster)  [unwired: 9 in]
  n195 = call <vilib>:"General Error Handler.vi"("type of dialog (OK msg:1)"=w6, "error in (no error)"=w5) -> ()  [unwired: 1 in, 13 out]
  n196 = local write "graph_update"(FALSE ("graph_update")) -> ()
  n197 = property on="Graphs T" class="WFChart (strict)"("YScale.ScaleFit"=u8 2 ("Y Scale.Scale Fit")) -> ()  [unwired: 2 in, 2 out]
  n198 = property on="мин." class="Str"("Disabled"=w25) -> (error out=w24:errorcluster)  [unwired: 2 in, 1 out]
  n199 = property on="часы" class="Str"(error in=w24, "Disabled"=w25) -> (error out=w23:errorcluster)  [unwired: 1 in, 1 out]
  n200 = invoke on="Добавить время" class="Ring (strict)" method="Reinit To Default"(error in=w23) -> (error out=w17:errorcluster)  [unwired: 2 in, 2 out]
  n201 = property on="Tab Control" class="TabCtl (strict)"() -> ("Pages"=w18:refnum<vi>[])  [unwired: 2 in, 2 out]
  n202 = invoke on="header?" class="Bool (strict)" method="Reinit To Default"(error in=w17) -> (error out=w22:errorcluster)  [unwired: 2 in, 2 out]
  n203 = invoke on="Graphs T" class="WFChart (strict)" method="Reinit To Default"() -> (error out=w13:errorcluster)  [unwired: 3 in, 2 out]
  n204 = Index Array(array=w18, index=1) -> (element=w19:refnum<vi>)
  n205 = property class="Page"(reference=w19, "PageEnb"=T6."Page Enabled" ("Page Enabled State")) -> ()  [unwired: 1 in, 2 out]
  n206 = property on="Расположение файла" class="Path"(error in=w22, "Disabled"=u8 2) -> ()  [unwired: 1 in, 2 out]
  n207 = property on="Graphs T" class="WFChart (strict)"(error in=w13, "Value"=dynamicdata [{"t0"=timestamp(3465273261.7246556 s since 1904-01-01), "dt"=1.0, "Y"=[0.1931097262457384]}, {"t0"=timestamp(3465273261.7246556 s since 1904-01-01), "dt"=1.0, "Y"=[0.3594116459482981]}, {"t0"=timestamp(3465273261.7246556 s since 1904-01-01), "dt"=1.0, "Y"=[0.8898205452798131]}, {"t0"=timestamp(3465273261.7246556 s since 1904-01-01), "dt"=1.0, "Y"=[0.747699236883661]}] ("Graphs")) -> (error out=w12:errorcluster)  [unwired: 1 in, 1 out]
  n208 = property on="Graphs T" class="WFChart (strict)"(error in=w12, "History Data"=dynamicdata[] []) -> (error out=w16:errorcluster)  [unwired: 1 in, 1 out]
  n209 = property on="Graphs T" class="WFChart (strict)"(error in=w16, "XScale.ScaleFit"=u8 0 ("Y Scale.Scale Fit")) -> ()  [unwired: 1 in, 2 out]
  n210 = event shown="[0] \"stop\": Value Change" {
    selector: _ -> [_]
    dyn-events: _ -> [_]
    timeout: _ -> [_]
    event "stop": Value Change {
      w381 = FALSE ("Запись в файл")
      n211 = event-data() -> ()  [unwired: 1 in, 1 out]
      n212 = local read "con ID"() -> (w378:refnum<k5>)
      n213 = property on="Запись в файл" class="Bool (strict)"("Value"=FALSE ("Запись в файл")) -> ()  [unwired: 2 in, 2 out]
      n214 = TCP Close Connection(connection ID=w378) -> (error out=w384:errorcluster)  [unwired: 1 in, 2 out]
      n215 = flat-sequence {
        tunnel: [w387] -> w383
        tunnel: w384 -> [w387]
        frame #0 {
          n216 = Wait (ms)(milliseconds to wait=u32 50) -> ()  [unwired: 1 out]
        }
      }
      n217 = local read "refnum out"() -> (w380:refnum<file>)
      n218 = Close File(refnum=w380, error in=w383) -> (error out=w379:errorcluster)  [unwired: 1 out]
      n219 = property on="Запись в файл" class="Bool (strict)"(error in=w379, "Value"=w381) -> (error out=w377:errorcluster)  [unwired: 1 in, 1 out]
      n220 = local write item#8(w381) -> ()
      n221 = flat-sequence {
        tunnel: w377 -> [w386]
        tunnel: [w386] -> _
        frame #0 {
          n222 = Stop(stop? (T)=TRUE) -> ()
        }
      }
    }
  }
  "счетчик" <- u32 0 ("счетчик")
